vi "Read FIRE U16 files (SubVI).vi"(11 "file path (use dialog)":path) -> (3 "Array":u16[][][](array[numeric]))   [LabVIEW 2018]
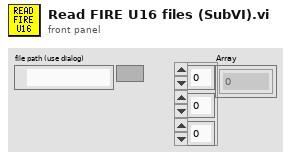
[diagram p1: front panel]
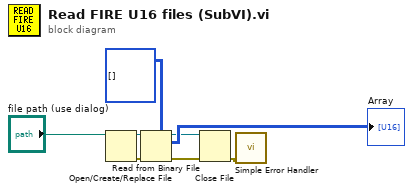
[diagram p0: block diagram]
diagram:
  n1 = Open/Create/Replace File(file path (use dialog)="file path (use dialog)") -> (refnum out=w6:refnum<file>, error out=w5:errorcluster)  [unwired: 5 in, 1 out]
  n2 = Read from Binary File(5:u16[][][] [], 8:w5, 11:w6) -> (0:w3:errorcluster, 2:→"Array":u16[][][], 3:w2:refnum<file>)  [unwired: 3 in, 1 out]
  n3 = Close File(refnum=w2, error in=w3) -> (error out=w4:errorcluster)  [unwired: 1 out]
  n4 = call <vilib>:"Simple Error Handler.vi"("error in (no error)"=w4) -> ()  [unwired: 4 in, 5 out]
